vi "XLP80_CAN_ReadFiles.vi"(7 "Function":string, 8 "error in":errorcluster) -> (0 "error out":errorcluster, 2 "Canceled":bool, 3 "variant":variant)   [LabVIEW 2021]
uses:
  XLP80_Globals/XLP80_CAN_Globals.vi
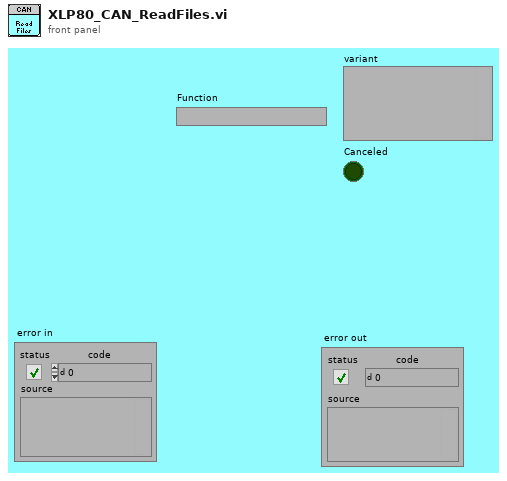
[diagram p1: front panel]
types:
  T1 = cluster{"Signal Name":string[], "Description":string[], "Unit":string[], "Min":dbl[], "Max":dbl[], "TestmodeA":bool[], "LogEnable":bool[]}
  T2 = cluster{"Signal Name":string[], "Description":string[], "Unit":string[], "Min":dbl[], "Max":dbl[], "HV & Software":bool[], "Basis Funktion":bool[], "Power Management":bool[], "OperationMode":bool[], "Shutdown":bool[], "Alarm":bool[], "LogEnable":bool[]}
  T3 = cluster{"Signal Name":string[], "Description":string[], "Unit":string[], "Default":dbl[], "Min":dbl[], "Max":dbl[], "TestmodeA":bool[], "LogEnable":bool[]}
  T4 = cluster{"Signal Name":string[], "Description":string[], "Unit":string[], "Default":dbl[], "Min":dbl[], "Max":dbl[], "Preconditions":bool[], "HV & Software":bool[], "Basis Funktion":bool[], "Power Management":bool[], "OperationMode":bool[], "Shutdown":bool[], "Alarm":bool[], "LogEnable":bool[]}
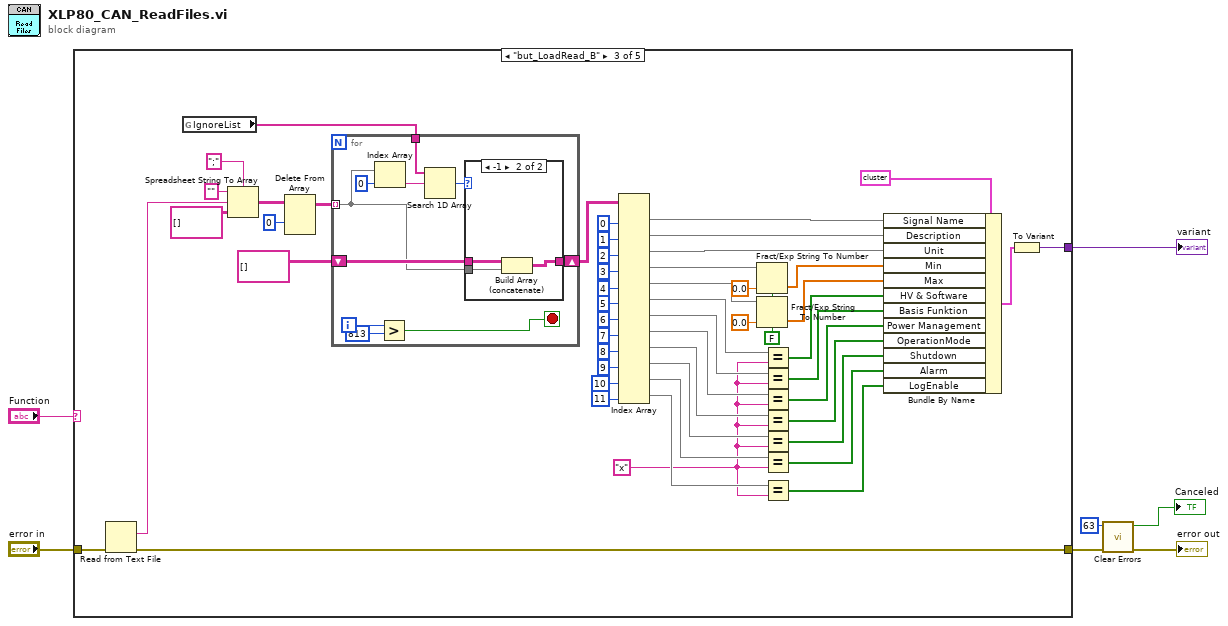
[diagram p0: block diagram]
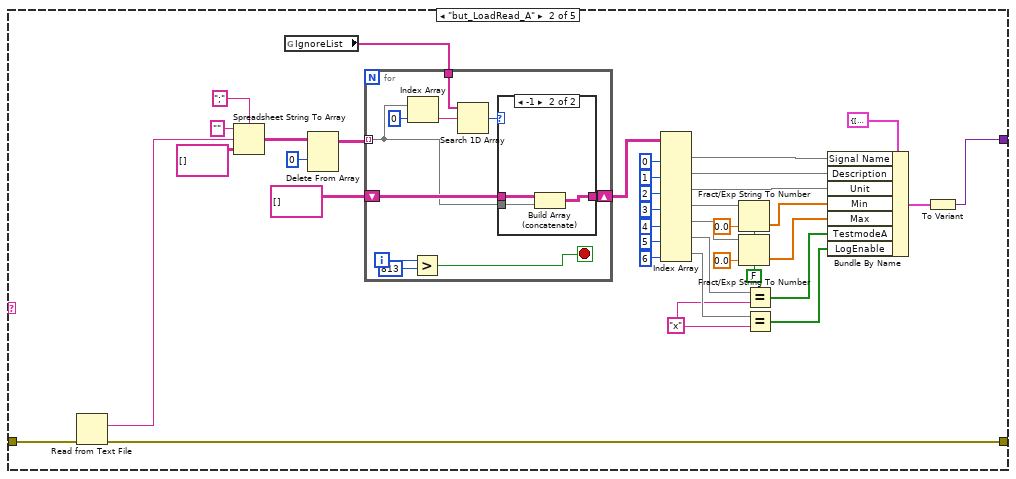
[diagram p3: hidden frame]
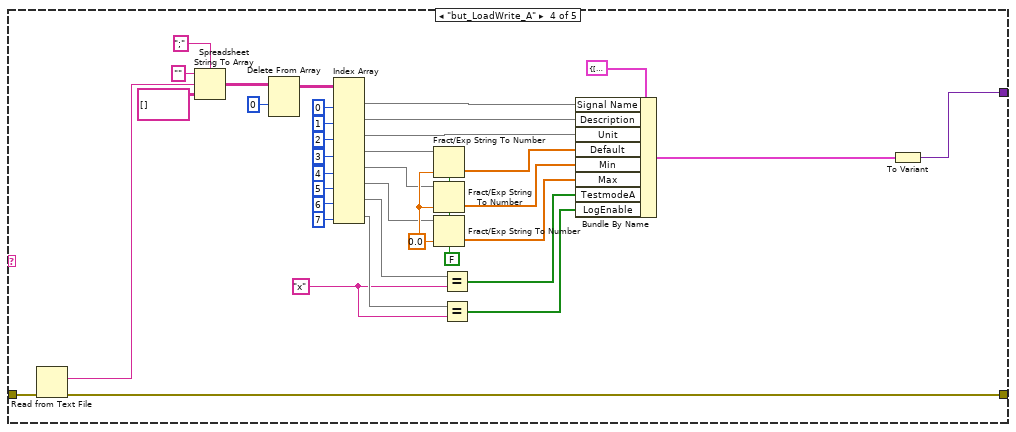
[diagram p6: hidden frame]
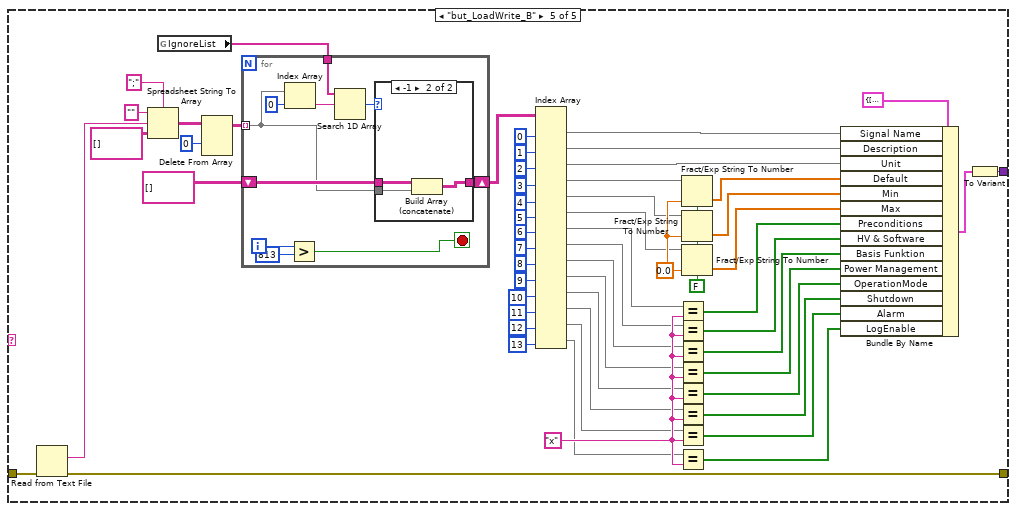
[diagram p7: hidden frame]
diagram:
  n1 = case shown="\"but_LoadRead_B\"" "Function" {
    tunnel: "error in" -> [w8 w26 w92 w137 w196]
    tunnel: [w8 w25 w91 w136 w195] -> w5
    tunnel: [_ w24 w90 w138 w197] -> w4
    frame Default {
    }
    frame "but_LoadRead_A" {
      w10 = "x" ("format string")
      w27 = FALSE ("use system decimal point (T)")
      n2 = Read from Text File(error in=w26) -> (text=w45:string, error out=w25:errorcluster)  [unwired: 3 in, 2 out]
      n3 = Spreadsheet String To Array(delimiter (Tab)=";", format string="", spreadsheet string=w45, array type (2D Dbl)=string[][] []) -> (array=w37:string[][])
      n4 = global read "XLP80_CAN_Globals.vi" "IgnoreList"() -> (w19:string[])
      n5 = Delete From Array(array=w37, index (row)=0) -> (array with subset deleted=w18:string[][])  [unwired: 2 in, 1 out]
      n6 = for {
        tunnel: w18 -> [w49] mode=indexing
        tunnel: w19 -> [w53]
        shift-right: [w50] -> w17
        shift-left: string[][] [] ("array w/ subset deleted") -> [w51]
        i -> [w48]
        stop <- w46 stop-if-true
        n7 = Index Array(array=w49, index=0) -> (element=w54:string)
        n8 = Greater?(x=w48, y=813) -> (0:w46:bool)
        n9 = Search 1D Array(1D array=w53, element=w54) -> (index of element=w52:i32)  [unwired: 1 in]
        n10 = case shown="-1" w52 {
          tunnel: w51 -> [w56 w59]
          tunnel: [w56 w57] -> w50
          tunnel: w49 -> [_ w58]
          frame Default {
          }
          frame -1 {
            n11 = Build Array (concatenate)(w59, w58) -> (w57:string[][])
          }
        }
      }
      n12 = Index Array(array=w17, index (col) #1=0 ("disabled index (col)"), index (col) #2=1 ("index (col)"), index (col) #3=2 ("index (col)"), index (col) #4=3 ("index (col)"), index (col) #5=4 ("index (col)"), index (col) #6=5 ("index (col)"), index (col) #7=6 ("index (col)")) -> (element #1=w16:string[], element #2=w40:string[], element #3=w39:string[], element #4=w33:string[], element #5=w29:string[], element #6=w13:string[], element #7=w11:string[])  [unwired: 7 in]
      n13 = Fract/Exp String To Number(use system decimal point (T)=w27, string=w33, default (0 dbl)=0.0 ("default (0 DBL)")) -> (number=w32:dbl[])  [unwired: 1 in, 1 out]
      n14 = Fract/Exp String To Number(use system decimal point (T)=w27, string=w29, default (0 dbl)=0.0 ("default (0 DBL)")) -> (number=w28:dbl[])  [unwired: 1 in, 1 out]
      n15 = Equal?(x=w13, y=w10) -> (x = y?=w12:bool[])
      n16 = Equal?(x=w11, y=w10) -> (x = y?=w9:bool[])
      n17 = Bundle By Name(cluster=T1 {"Signal Name"=[], "Description"=[], "Unit"=[], "Min"=[], "Max"=[], "TestmodeA"=[], "LogEnable"=[]} ("Settings_CANRead_Testmode_A"), "Signal Name"=w16, "Description"=w40, "Unit"=w39, "Min"=w32, "Max"=w28, "TestmodeA"=w12, "LogEnable"=w9) -> (w22:T1)
      n18 = To Variant(anything=w22) -> (Variant=w24:variant)
    }
    frame "but_LoadRead_B" {
      w61 = "x" ("format string")
      w93 = FALSE ("use system decimal point (T)")
      n19 = Read from Text File(error in=w92) -> (text=w111:string, error out=w91:errorcluster)  [unwired: 3 in, 2 out]
      n20 = global read "XLP80_CAN_Globals.vi" "IgnoreList"() -> (w86:string[])
      n21 = Spreadsheet String To Array(delimiter (Tab)=";", format string="", spreadsheet string=w111, array type (2D Dbl)=string[][] []) -> (array=w103:string[][])
      n22 = Delete From Array(array=w103, index (row)=0) -> (array with subset deleted=w89:string[][])  [unwired: 2 in, 1 out]
      n23 = for {
        tunnel: w89 -> [w115] mode=indexing
        tunnel: w86 -> [w119]
        shift-right: [w116] -> w87
        shift-left: string[][] [] ("array w/ subset deleted") -> [w117]
        i -> [w114]
        stop <- w112 stop-if-true
        n24 = Index Array(array=w115, index=0) -> (element=w120:string)
        n25 = Greater?(x=w114, y=813) -> (0:w112:bool)
        n26 = Search 1D Array(1D array=w119, element=w120) -> (index of element=w118:i32)  [unwired: 1 in]
        n27 = case shown="-1" w118 {
          tunnel: w117 -> [w122 w125]
          tunnel: [w122 w123] -> w116
          tunnel: w115 -> [_ w124]
          frame Default {
          }
          frame -1 {
            n28 = Build Array (concatenate)(w125, w124) -> (w123:string[][])
          }
        }
      }
      n29 = Index Array(array=w87, index (col) #1=0 ("disabled index (col)"), index (col) #2=1 ("index (col)"), index (col) #3=2 ("index (col)"), index (col) #4=3 ("index (col)"), index (col) #5=4 ("index (col)"), index (col) #6=5 ("index (col)"), index (col) #7=6 ("index (col)"), index (col) #8=7 ("index (col)"), index (col) #9=8 ("index (col)"), index (col) #10=9 ("index (col)"), index (col) #11=10 ("index (col)"), index (col) #12=11 ("index (col)")) -> (element #1=w64:string[], element #2=w106:string[], element #3=w105:string[], element #4=w99:string[], element #5=w95:string[], element #6=w83:string[], element #7=w76:string[], element #8=w74:string[], element #9=w72:string[], element #10=w70:string[], element #11=w68:string[], element #12=w62:string[])  [unwired: 12 in]
      n30 = Fract/Exp String To Number(use system decimal point (T)=w93, string=w99, default (0 dbl)=0.0 ("default (0 DBL)")) -> (number=w98:dbl[])  [unwired: 1 in, 1 out]
      n31 = Fract/Exp String To Number(use system decimal point (T)=w93, string=w95, default (0 dbl)=0.0 ("default (0 DBL)")) -> (number=w94:dbl[])  [unwired: 1 in, 1 out]
      n32 = Equal?(x=w83, y=w61) -> (x = y?=w82:bool[])
      n33 = Equal?(x=w76, y=w61) -> (x = y?=w75:bool[])
      n34 = Equal?(x=w74, y=w61) -> (x = y?=w73:bool[])
      n35 = Equal?(x=w72, y=w61) -> (x = y?=w71:bool[])
      n36 = Equal?(x=w70, y=w61) -> (x = y?=w69:bool[])
      n37 = Equal?(x=w68, y=w61) -> (x = y?=w67:bool[])
      n38 = Equal?(x=w62, y=w61) -> (x = y?=w60:bool[])
      n39 = Bundle By Name(cluster=T2 data[44510B] ("Settings_CANRead_Testmode_B"), "Signal Name"=w64, "Description"=w106, "Unit"=w105, "Min"=w98, "Max"=w94, "HV & Software"=w82, "Basis Funktion"=w75, "Power Management"=w73, "OperationMode"=w71, "Shutdown"=w69, "Alarm"=w67, "LogEnable"=w60) -> (w85:T2)
      n40 = To Variant(anything=w85) -> (Variant=w90:variant)
    }
    frame "but_LoadWrite_A" {
      w144 = FALSE ("use system decimal point (T)")
      w128 = "x" ("format string")
      w146 = 0.0 ("default (0 DBL)")
      n41 = Read from Text File(error in=w137) -> (text=w159:string, error out=w136:errorcluster)  [unwired: 3 in, 2 out]
      n42 = Spreadsheet String To Array(delimiter (Tab)=";", format string="", spreadsheet string=w159, array type (2D Dbl)=string[][] []) -> (array=w160:string[][])
      n43 = Delete From Array(array=w160, index (row)=0) -> (array with subset deleted=w161:string[][])  [unwired: 2 in, 1 out]
      n44 = Index Array(array=w161, index (col) #1=0 ("disabled index (col)"), index (col) #2=1 ("index (col)"), index (col) #3=2 ("index (col)"), index (col) #4=3 ("index (col)"), index (col) #5=4 ("index (col)"), index (col) #6=5 ("index (col)"), index (col) #7=6 ("index (col)"), index (col) #8=7 ("index (col)")) -> (element #1=w133:string[], element #2=w158:string[], element #3=w157:string[], element #4=w145:string[], element #5=w143:string[], element #6=w142:string[], element #7=w130:string[], element #8=w129:string[])  [unwired: 8 in]
      n45 = Fract/Exp String To Number(use system decimal point (T)=w144, string=w145, default (0 dbl)=w146) -> (number=w141:dbl[])  [unwired: 1 in, 1 out]
      n46 = Fract/Exp String To Number(use system decimal point (T)=w144, string=w143, default (0 dbl)=w146) -> (number=w140:dbl[])  [unwired: 1 in, 1 out]
      n47 = Fract/Exp String To Number(use system decimal point (T)=w144, string=w142, default (0 dbl)=w146) -> (number=w139:dbl[])  [unwired: 1 in, 1 out]
      n48 = Equal?(x=w130, y=w128) -> (x = y?=w127:bool[])
      n49 = Equal?(x=w129, y=w128) -> (x = y?=w126:bool[])
      n50 = Bundle By Name(cluster=T3 {"Signal Name"=[], "Description"=[], "Unit"=[], "Default"=[], "Min"=[], "Max"=[], "TestmodeA"=[], "LogEnable"=[]} ("Settings_CANWrite_Testmode_A"), "Signal Name"=w133, "Description"=w158, "Unit"=w157, "Default"=w141, "Min"=w140, "Max"=w139, "TestmodeA"=w127, "LogEnable"=w126) -> (w134:T3)
      n51 = To Variant(anything=w134) -> (Variant=w138:variant)
    }
    frame "but_LoadWrite_B" {
      w173 = "x" ("format string")
      w203 = FALSE ("use system decimal point (T)")
      w205 = 0.0 ("default (0 DBL)")
      n52 = Read from Text File(error in=w196) -> (text=w217:string, error out=w195:errorcluster)  [unwired: 3 in, 2 out]
      n53 = Spreadsheet String To Array(delimiter (Tab)=";", format string="", spreadsheet string=w217, array type (2D Dbl)=string[][] []) -> (array=w218:string[][])
      n54 = global read "XLP80_CAN_Globals.vi" "IgnoreList"() -> (w191:string[])
      n55 = Delete From Array(array=w218, index (row)=0) -> (array with subset deleted=w190:string[][])  [unwired: 2 in, 1 out]
      n56 = for {
        tunnel: w190 -> [w222] mode=indexing
        tunnel: w191 -> [w226]
        shift-right: [w223] -> w189
        shift-left: string[][] [] ("array w/ subset deleted") -> [w224]
        i -> [w221]
        stop <- w219 stop-if-true
        n57 = Index Array(array=w222, index=0) -> (element=w227:string)
        n58 = Greater?(x=w221, y=813) -> (0:w219:bool)
        n59 = Search 1D Array(1D array=w226, element=w227) -> (index of element=w225:i32)  [unwired: 1 in]
        n60 = case shown="-1" w225 {
          tunnel: w224 -> [w229 w232]
          tunnel: [w229 w230] -> w223
          tunnel: w222 -> [_ w231]
          frame Default {
          }
          frame -1 {
            n61 = Build Array (concatenate)(w232, w231) -> (w230:string[][])
          }
        }
      }
      n62 = Index Array(array=w189, index (col) #1=0 ("disabled index (col)"), index (col) #2=1 ("index (col)"), index (col) #3=2 ("index (col)"), index (col) #4=3 ("index (col)"), index (col) #5=4 ("index (col)"), index (col) #6=5 ("index (col)"), index (col) #7=6 ("disabled index (col)"), index (col) #8=7 ("index (col)"), index (col) #9=8 ("index (col)"), index (col) #10=9 ("index (col)"), index (col) #11=10 ("index (col)"), index (col) #12=11 ("index (col)"), index (col) #13=12 ("index (col)"), index (col) #14=13 ("index (col)")) -> (element #1=w176:string[], element #2=w216:string[], element #3=w215:string[], element #4=w204:string[], element #5=w202:string[], element #6=w201:string[], element #7=w170:string[], element #8=w168:string[], element #9=w167:string[], element #10=w166:string[], element #11=w165:string[], element #12=w164:string[], element #13=w163:string[], element #14=w162:string[])  [unwired: 14 in]
      n63 = Equal?(x=w170, y=w173) -> (x = y?=w169:bool[])
      n64 = Equal?(x=w168, y=w173) -> (x = y?=w182:bool[])
      n65 = Equal?(x=w167, y=w173) -> (x = y?=w181:bool[])
      n66 = Equal?(x=w166, y=w173) -> (x = y?=w180:bool[])
      n67 = Equal?(x=w165, y=w173) -> (x = y?=w179:bool[])
      n68 = Equal?(x=w164, y=w173) -> (x = y?=w178:bool[])
      n69 = Equal?(x=w163, y=w173) -> (x = y?=w177:bool[])
      n70 = Equal?(x=w162, y=w173) -> (x = y?=w174:bool[])
      n71 = Fract/Exp String To Number(use system decimal point (T)=w203, string=w204, default (0 dbl)=w205) -> (number=w200:dbl[])  [unwired: 1 in, 1 out]
      n72 = Fract/Exp String To Number(use system decimal point (T)=w203, string=w202, default (0 dbl)=w205) -> (number=w199:dbl[])  [unwired: 1 in, 1 out]
      n73 = Fract/Exp String To Number(use system decimal point (T)=w203, string=w201, default (0 dbl)=w205) -> (number=w198:dbl[])  [unwired: 1 in, 1 out]
      n74 = Bundle By Name(cluster=T4 {"Signal Name"=[], "Description"=[], "Unit"=[], "Default"=[], "Min"=[], "Max"=[], "Preconditions"=[], "HV & Software"=[], "Basis Funktion"=[], "Power Management"=[], "OperationMode"=[], "Shutdown"=[], "Alarm"=[], "LogEnable"=[]} ("Settings_CANWrite_Testmode_B"), "Signal Name"=w176, "Description"=w216, "Unit"=w215, "Default"=w200, "Min"=w199, "Max"=w198, "Preconditions"=w169, "HV & Software"=w182, "Basis Funktion"=w181, "Power Management"=w180, "OperationMode"=w179, "Shutdown"=w178, "Alarm"=w177, "LogEnable"=w174) -> (w194:T4)
      n75 = To Variant(anything=w194) -> (Variant=w197:variant)
    }
  }
  "variant" <- w4
  n76 = call <vilib>:"Clear Errors.vi"("error in (no error)"=w5, "specific error code to clear (0: all)"=63) -> ("error out"=→"error out":errorcluster, "specific error cleared?"=→"Canceled":bool)  [unwired: 4 in]
